vi "Set Exp to test_Floor and Roof.vi"(0 "Test Information":T3={"Exp Name"="Cold Switching", "Lot"="0233A", "Wafer"="15", "Die Type"="L22", "Die X "="6", "Die Y"="8", "Exp"="1", "Die X_Y"="8"}, 5 "Experiments":T1={"Exp 1"={"Floor_Sweep_Stop_V"=36.0, "Resistance Threshold"=1.0, "Floor_Sweep_Start_V"=36.0, "Floor_Sweep_Step_V"=1.0, "Roof_Sweep_Stop_V"=36.0, "Roof_Sweep_Start_V"=36.0, "Roof_Sweep_Step_V"=1.0, "Meas Type"=enum."Floor", "Experiment Name"=""}, "Exp 2"={"Floor_Sweep_Stop_V"=36.0, "Resistance Threshold"=1.0, "Floor_Sweep_Start_V"=36.0, "Floor_Sweep_Step_V"=1.0, "Roof_Sweep_Stop_V"=36.0, "Roof_Sweep_Start_V"=36.0, "Roof_Sweep_Step_V"=1.0, "Meas Type"=enum."Floor", "Experiment Name"=""}, "Exp 3"={"Floor_Sweep_Stop_V"=36.0, "Resistance Threshold"=1.0, "Floor_Sweep_Start_V"=36.0, "Floor_Sweep_Step_V"=1.0, "Roof_Sweep_Stop_V"=36.0, "Roof_Sweep_Start_V"=36.0, "Roof_Sweep_Step_V"=1.0, "Meas Type"=enum."Floor", "Experiment Name"=""}, "Exp 4"={"Floor_Sweep_Stop_V"=36.0, "Resistance Threshold"=1.0, "Floor_Sweep_Start_V"=36.0, "Floor_Sweep_Step_V"=1.0, "Roof_Sweep_Stop_V"=36.0, "Roof_Sweep_Start_V"=36.0, "Roof_Sweep_Step_V"=1.0, "Meas Type"=enum."Floor", "Experiment Name"=""}}, 11 "Error In":errorcluster) -> (4 "Selected Exp Settings":T2={"Floor_Sweep_Stop_V"=36.0, "Resistance Threshold"=1.0, "Floor_Sweep_Start_V"=36.0, "Floor_Sweep_Step_V"=1.0, "Roof_Sweep_Stop_V"=36.0, "Roof_Sweep_Start_V"=36.0, "Roof_Sweep_Step_V"=1.0, "Meas Type"=enum."Floor", "Experiment Name"=""}, 6 "Test Information Out":T3={"Exp Name"="Cold Switching", "Lot"="0233A", "Wafer"="15", "Die Type"="L22", "Die X "="6", "Die Y"="8", "Exp"="1", "Die X_Y"="8"}, 15 "Error Out":errorcluster)   [LabVIEW 2013]
uses:
  Controls/Test Information.ctl
  Controls/Individual User Inputs_Floor and Roof.ctl
  Controls/Multiple Exp Setup_Floor and Roof.ctl
panel:
  # "Test Settings"
  # "Calculation Settings"
  # "Test Settings"
  # "Calculation Settings"
  # "Test Settings"
  # "Calculation Settings"
  # "Test Settings"
  # "Calculation Settings"
  # "Test Settings"
  # "Calculation Settings"
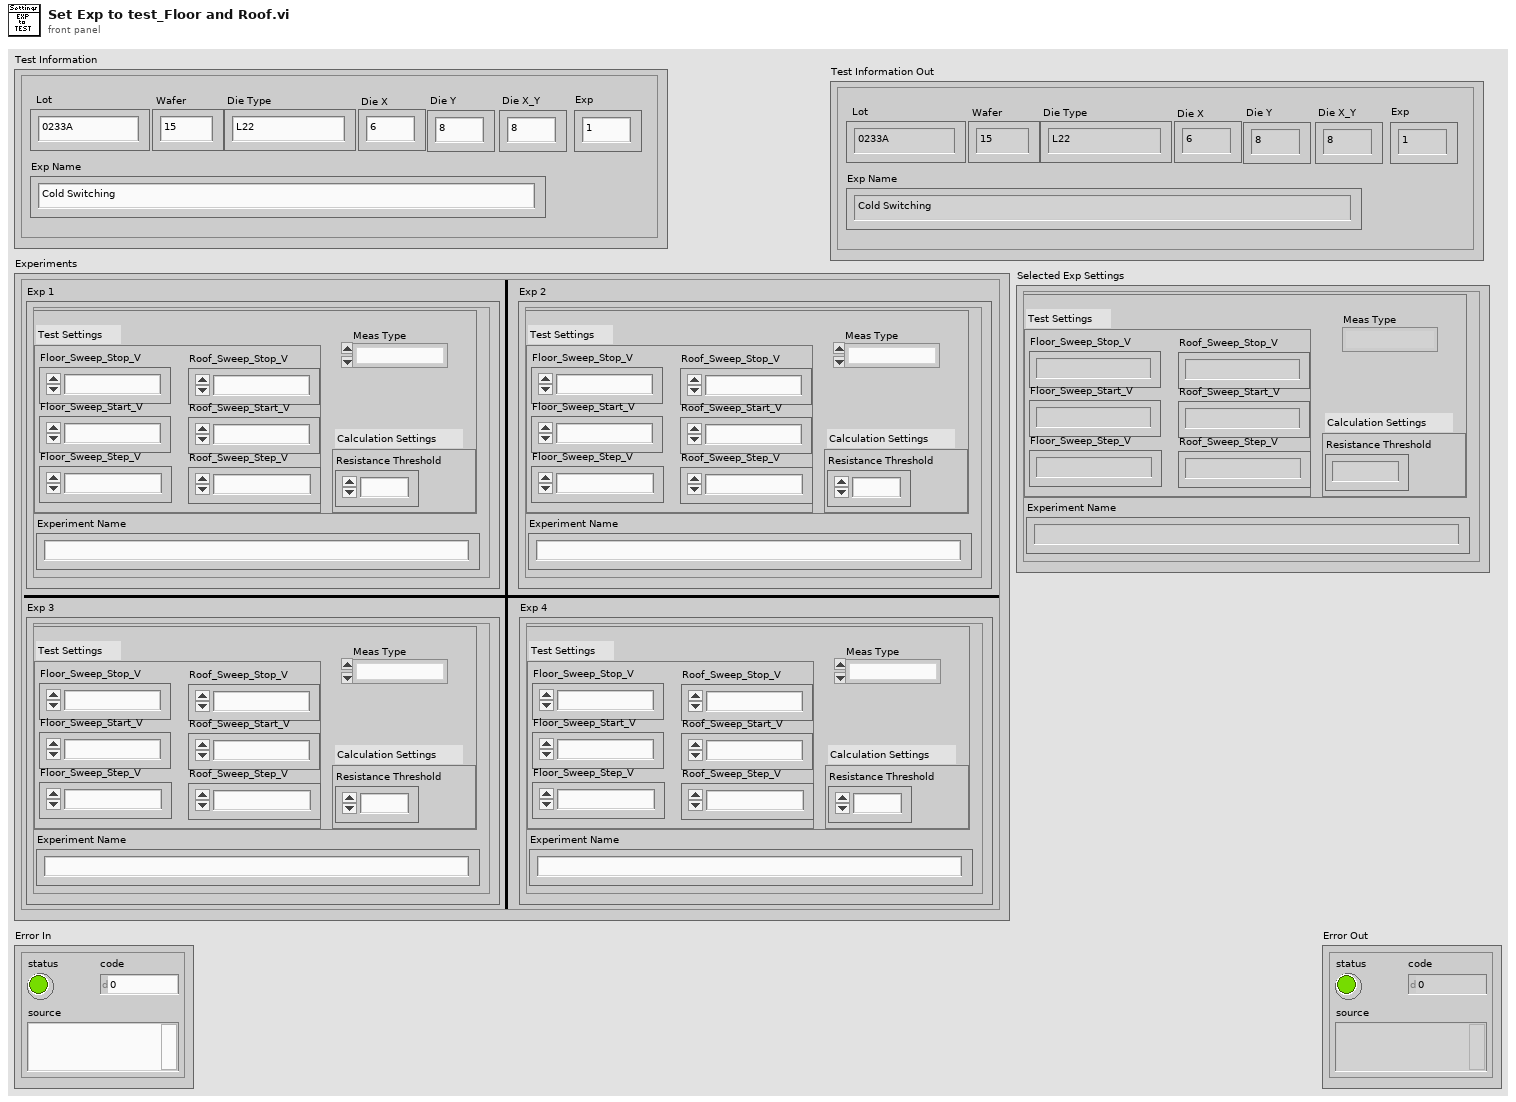
[diagram p1: front panel]
types:
  T1 = typedef "Multiple Exp Setup_Floor and Roof.ctl" = cluster{"Exp 1":T2, "Exp 2":T2, "Exp 3":T2, "Exp 4":T2}
  T2 = typedef "Individual User Inputs_Floor and Roof.ctl" = cluster{"Floor_Sweep_Stop_V":dbl, "Resistance Threshold":dbl, "Floor_Sweep_Start_V":dbl, "Floor_Sweep_Step_V":dbl, "Roof_Sweep_Stop_V":dbl, "Roof_Sweep_Start_V":dbl, "Roof_Sweep_Step_V":dbl, "Meas Type":enum16{"Floor", "Roof", "Floor and Roof"}, "Experiment Name":string}
  T3 = typedef "Test Information.ctl" = cluster{"Exp Name":string, "Lot":string, "Wafer":string, "Die Type":string, "Die X ":string, "Die Y":string, "Exp":string, "Die X_Y":string}
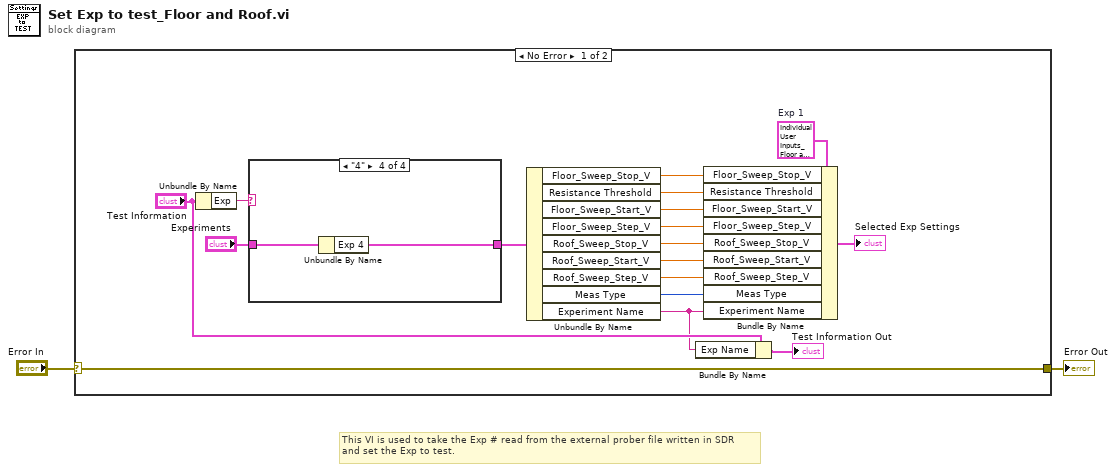
[diagram p0: block diagram]
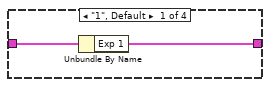
[diagram p2: hidden frame]
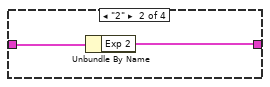
[diagram p3: hidden frame]
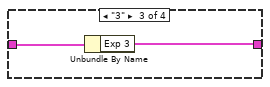
[diagram p4: hidden frame]
diagram:
  # "This VI is used to take the Exp # read from the external prober file written in SDR\nand set the Exp to test."
  n1 = case shown="No Error" "Error In" {
    selector: "Error In" -> [w18 w28]
    tunnel: [w18 w28] -> w1
    frame No Error {
      w16 = T2 {"Floor_Sweep_Stop_V"=36.0, "Resistance Threshold"=1.0, "Floor_Sweep_Start_V"=36.0, "Floor_Sweep_Step_V"=1.0, "Roof_Sweep_Stop_V"=36.0, "Roof_Sweep_Start_V"=36.0, "Roof_Sweep_Step_V"=1.0, "Meas Type"=enum."Floor", "Experiment Name"=""}  # Exp 1
      n2 = Unbundle By Name("Test Information") -> ("Exp"=w19:string)
      n3 = case shown="\"4\"" w19 {
        tunnel: [w20 w23 w25 w27] -> w12
        tunnel: "Experiments" -> [w21 w22 w24 w26]
        frame "1", Default {
          n4 = Unbundle By Name(w21) -> ("Exp 1"=w20:T2)
        }
        frame "2" {
          n5 = Unbundle By Name(w22) -> ("Exp 2"=w23:T2)
        }
        frame "3" {
          n6 = Unbundle By Name(w24) -> ("Exp 3"=w25:T2)
        }
        frame "4" {
          n7 = Unbundle By Name(w26) -> ("Exp 4"=w27:T2)
        }
      }
      n8 = Unbundle By Name(w12) -> ("Floor_Sweep_Stop_V"=w11:dbl, "Resistance Threshold"=w10:dbl, "Floor_Sweep_Start_V"=w9:dbl, "Floor_Sweep_Step_V"=w8:dbl, "Roof_Sweep_Stop_V"=w7:dbl, "Roof_Sweep_Start_V"=w6:dbl, "Roof_Sweep_Step_V"=w5:dbl, "Meas Type"=w4:enum16{"Floor", "Roof", "Floor and Roof"}, "Experiment Name"=w3:string)
      n9 = Bundle By Name(cluster="Test Information", "Exp Name"=w3) -> (→"Test Information Out":T3)
      n10 = Bundle By Name(cluster=w16, "Floor_Sweep_Stop_V"=w11, "Resistance Threshold"=w10, "Floor_Sweep_Start_V"=w9, "Floor_Sweep_Step_V"=w8, "Roof_Sweep_Stop_V"=w7, "Roof_Sweep_Start_V"=w6, "Roof_Sweep_Step_V"=w5, "Meas Type"=w4, "Experiment Name"=w3) -> (→"Selected Exp Settings":T2)
    }
    frame Error {
    }
  }
  "Error Out" <- w1
